vi "Begin.vi"(8 "error in":errorcluster) -> (0 "error out":errorcluster)   [LabVIEW 2015]
doc: "Called before other user functions, this VI is expected to open initial I/O refnums, load in file data, and do all program initialization. Notice that the <B>error out</B> terminal is simply used for data flow. Wiring it to other structures or subVIs ensures that this VI runs first."
uses:
  <vilib>/Rock Robotics/WPI/SafetyOutput/WPI_SafetyOutputConfigMenu.ctl
  <vilib>/Rock Robotics/WPI/DriverStation/WPI_DriverStationRobotMode2.ctl
  <vilib>/Rock Robotics/WPI/Joystick/WPI_JoystickDeviceEnum.ctl
  <vilib>/Rock Robotics/SystemInterfaces/DIO/FPGA_DIOPWMChannel.ctl
  <vilib>/Rock Robotics/SystemInterfaces/AI/FPGA_AIGyroChannel.ctl
  Robot Global Data.vi
  <vilib>/Rock Robotics/Network Tables/NT Write String Array.vi
  <vilib>/Rock Robotics/WPI/MotorControl/WPI_MotorControlOpen Talon.vi
  <vilib>/Rock Robotics/WPI/RobotDrive/WPI_RobotDriveOpen4MotorWithExistingMotors.vi
  <vilib>/Rock Robotics/WPI/MotorControl/WPI_MotorControlOpen VictorSP.vi
  <vilib>/Rock Robotics/WPI/RobotDrive/WPI_RobotDriveOpen2MotorWithExistingMotors.vi
  <vilib>/Rock Robotics/WPI/Switch/WPI_SwitchOpenLimit.vi
  <vilib>/Rock Robotics/WPI/MotorControl/WPI_MotorControlOpen SPARK.vi
  <vilib>/Rock Robotics/WPI/MotorControl/WPI_MotorControlOpenCANTalonSRX.vi
  <vilib>/Rock Robotics/WPI/Gyro/WPI_GyroAnalogOpen.vi
  <vilib>/Rock Robotics/Network Tables/NT Write String.vi
  <vilib>/Rock Robotics/SystemInterfaces/spilib/spi_bus.ctl
  <vilib>/Rock Robotics/SystemInterfaces/DIO/FPGA_DIOChannel.ctl
  <vilib>/Rock Robotics/WPI/CAN/TalonSRX/WPI_CANTalonSRX_APIControlMode.ctl
  ADI MXP IMU/ADI MXP IMU/FRC ADI MXP IMU.lvlib
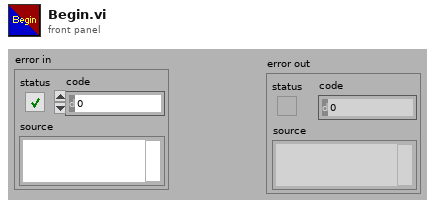
[diagram p1: front panel]
types:
  T1 = typedef "WPI_JoystickDeviceEnum.ctl" = enum16{"USB 0", "USB 1", "USB 2", "USB 3", "USB 4", "USB 5"}
  T2 = typedef "WPI_DriverStationRobotMode2.ctl" = enum16{"Autonomous Disabled", "Autonomous Enabled", "Teleop Disabled", "Teleop Enabled", "Disconnected", "Finish", "Test Disabled", "Test Enabled", "Emergency Stopped"}
  T3 = typedef "WPI_SafetyOutputConfigMenu.ctl" = enum16{"Enable", "Disable"}
  T4 = typedef "FPGA_DIOPWMChannel.ctl" = enum8{"PWM 0", "PWM 1", "PWM 2", "PWM 3", "PWM 4", "PWM 5", "PWM 6", "PWM 7", "PWM 8", "PWM 9", "PWM MXP 0", "PWM MXP 1", "PWM MXP 2", "PWM MXP 3", "PWM MXP 4", "PWM MXP 5", "PWM MXP 6", "PWM MXP 7", "PWM MXP 8", "PWM MXP 9", "Invalid"}
  T5 = typedef "WPI_MotorControlDeviceRef.ctl" = cluster{"DeviceStatus":errorcluster, "Type":T6, "PWM":cluster{"PWM Channel":T4, "DeadBand":T7}, "CAN":cluster{"Device Number":u8, "Control Mode":T8, "Semaphore":T9, "Max Vout":dbl, "TalonSRX Control Mode":T10}, "Invert":bool}
  T6 = typedef "WPI_MotorControlType.ctl" = enum16{"PWM", "CAN", "CANTalonSRX"}
  T7 = typedef "WPI_PWMDeadband.ctl" = cluster{"Name":string, "maxPositivePwm":i32, "minPositivePwm":i32, "centerPwm":i32, "maxNegativePwm":i32, "minNegativePwm":i32, "angularRange":u16}
  T8 = typedef "WPI_CANJaguar_ControlMode.ctl" = enum8{"Percent VBus", "Current", "Speed", "Position", "Voltage"}
  T9 = typedef "Semaphore RefNum" = refnum<k1>
  T10 = typedef "WPI_CANTalonSRX_APIControlMode.ctl" = enum8{"Percent VBus", "Speed", "Position", "Slave", "Unchanged / Invalid", "Voltage Compensation", "Current", "Motion Profile"}
  T11 = typedef "WPI_RobotDriveDevRef.ctl" = cluster{"DevStatus":errorcluster, "Motors[]":T5[], "Square Inputs":bool, "Max Output":dbl}
  T12 = typedef "WPI_JoystickDevRef.ctl" = cluster{"Device":T1}
  T13 = typedef "FPGA_DIOChannel.ctl" = enum8{"DIO 0", "DIO 1", "DIO 2", "DIO 3", "DIO 4", "DIO 5", "DIO 6", "DIO 7", "DIO 8", "DIO 9", "DIO MXP 0", "DIO MXP 1", "DIO MXP 2", "DIO MXP 3", "DIO MXP 4", "DIO MXP 5", "DIO MXP 6", "DIO MXP 7", "DIO MXP 8", "DIO MXP 9", "DIO MXP 10", "DIO MXP 11", "DIO MXP 12", "DIO MXP 13", "DIO MXP 14", "DIO MXP 15", "Invalid"}
  T14 = typedef "spi_bus.ctl" = enum16{"SPI On-Board, CS0", "SPI On-Board, CS1", "SPI On-Board, CS2", "SPI On-Board, CS3", "SPI MXP", "Invalid"}
  T15 = typedef "FPGA_AIGyroChannel.ctl" = enum8{"AI 0", "AI 1", "Invalid"}
  T16 = typedef "WPI_DigitalInputDevRef.ctl" = cluster{"DevStatus":errorcluster, "DIO Channel":T13}
  T17 = typedef "WPI_SwitchDevRef.ctl" = cluster{"DevStatus":errorcluster, "DIO Channel":T13, "CntIndex":T18, "Normally Closed":bool}
  T18 = typedef "FPGA_CounterCtrSystemIndex.ctl" = enum8{"Ctr 0", "Ctr 1", "Ctr 2", "Ctr 3", "Ctr 4", "Ctr 5", "Ctr 6", "Ctr 7", "Invalid"}
  T19 = typedef "FRC ADI MXP IMU.lvlib/WPI_AnalogDevicesIMUInterruptDevRef.ctl" = cluster{"SimpleGyroDevRef":T20, "InterruptRef":T21}
  T20 = typedef "FRC ADI MXP IMU.lvlib/WPI_AnalogDevicesIMUDevRef.ctl" = cluster{"DevStatus":errorcluster, "Handle":i32, "SPI Bus":T14, "Device Found":bool, "Sample Rate":dbl, "Device Ready":bool, "Yaw Axis":enum16{"X", "Y", "Z"}, "AHRS Algorithm":enum16{"Complementary", "Madgwick"}}
  T21 = typedef "WPI_InterruptRef.ctl" = cluster{"DevStatus":errorcluster, "InterruptIndex":T22}
  T22 = typedef "FPGA_InterruptIndex.ctl" = enum8{"0", "1", "2", "3", "4", "5", "6", "7", "Invalid"}
  T23 = typedef "WPI_GyroDevRef.ctl" = cluster{"DevStatus":errorcluster, "Analog Channel":T24, "Offset":dbl, "Gain (VoltsPerDegree/Second)":dbl, "Gyro Type":enum16{"Analog", "XRS450"}, "Handle":i32, "SPI Bus":T14, "Device Found":bool, "Sample Rate":dbl, "Calibrate On Open":bool}
  T24 = typedef "FPGA_AIChannel.ctl" = enum8{"AI 0", "AI 1", "AI 2", "AI 3", "AI MXP 0", "AI MXP 1", "AI MXP 2", "AI MXP 3", "Invalid"}
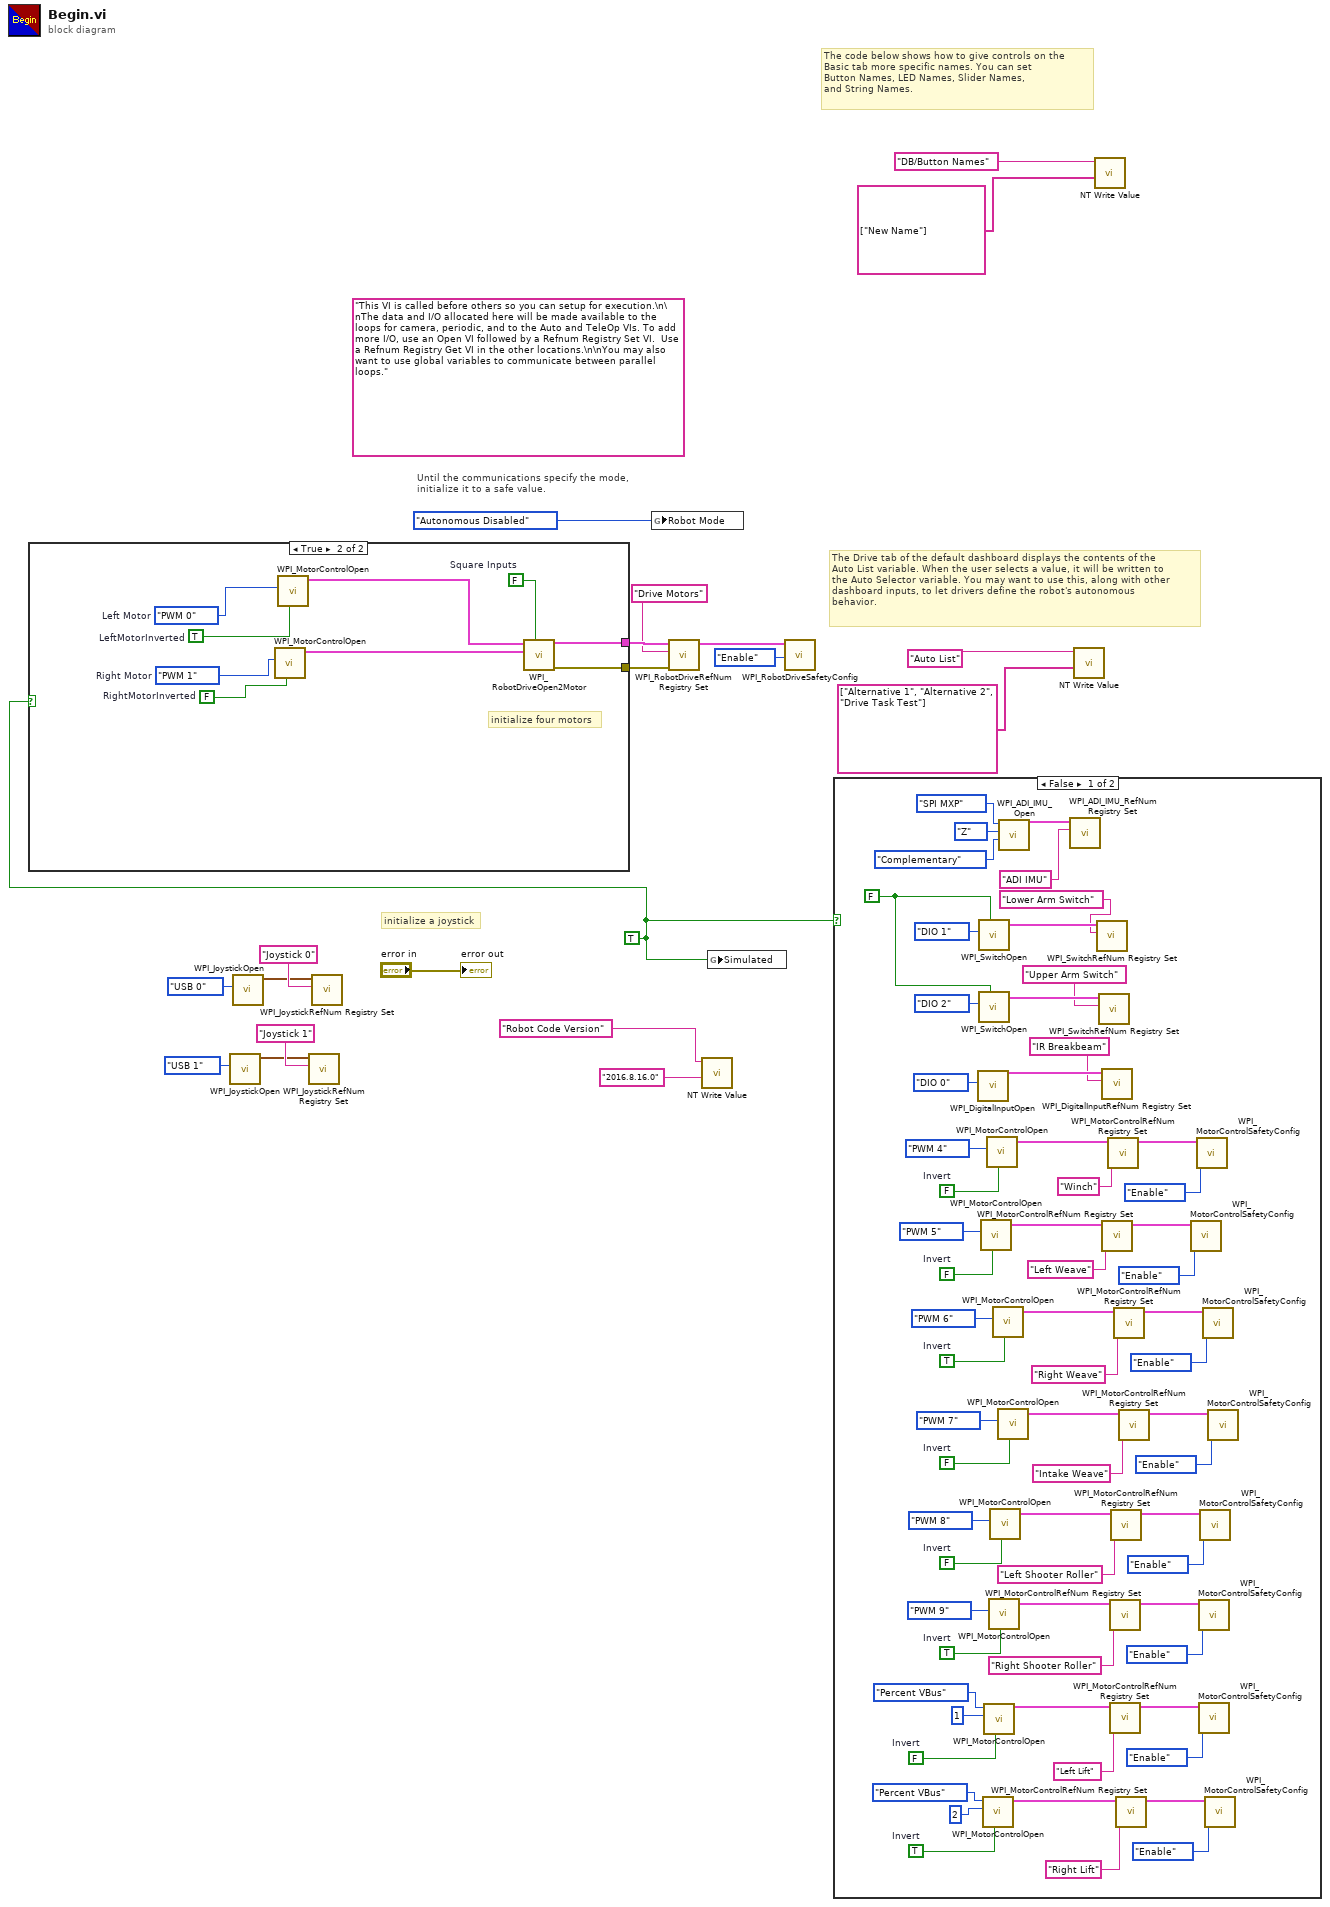
[diagram p0: block diagram]
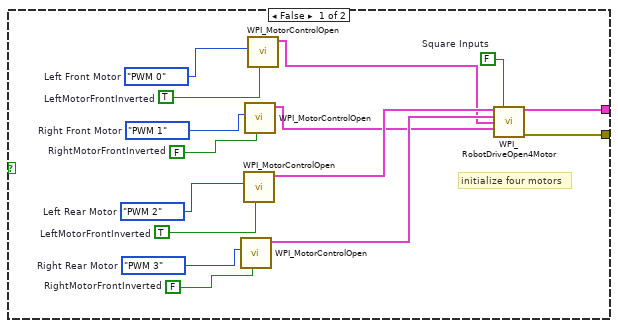
[diagram p2: hidden frame]
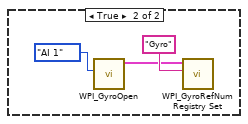
[diagram p3: hidden frame]
diagram:
  w1 = TRUE
  (unwired) "This VI is called before others so you can setup for execution.\n\nThe data and I/O allocated here will be made available to the loops for camera, periodic, and to the Auto and TeleOp VIs. To add more I/O, use an Open VI followed by a Refnum Registry Set VI.  Use a Refnum Registry Get VI in the other locations.\n\nYou may also want to use global variables to communicate between parallel loops."
  # "The Drive tab of the default dashboard displays the contents of the\nAuto List variable. When the user selects a value, it will be written to\nthe Auto Selector variable. You may want to use this, along with other\ndashboard inputs, to let drivers define the robot's autonomous\nbehavior."
  # "The code below shows how to give controls on the\nBasic tab more specific names. You can set\nButton Names, LED Names, Slider Names,\nand String Names."
  # "initialize a joystick"
  # "Until the communications specify the mode,\ninitialize it to a safe value."
  n1 = case shown="True" w1 {
    tunnel: [w35 w36] -> w20
    tunnel: [w34 w37] -> w18
    frame False {
      w27 = FPGA_DIOPWMChannel."PWM 3"  # Right Rear Motor
      w26 = FPGA_DIOPWMChannel."PWM 2"  # Left Rear Motor
      w25 = TRUE  # LeftMotorFrontInverted
      w28 = FALSE  # RightMotorFrontInverted
      w29 = FALSE  # Square Inputs
      w32 = FPGA_DIOPWMChannel."PWM 1"  # Right Front Motor
      w31 = FPGA_DIOPWMChannel."PWM 0"  # Left Front Motor
      w30 = TRUE  # LeftMotorFrontInverted
      w33 = FALSE  # RightMotorFrontInverted
      # "initialize four motors"
      n2 = call-poly <vilib>:"WPI_MotorControlOpen.vi"("Invert"=w28, "PWM Channel"=w27) -> ("MotorControlDeviceRef"=w23:T5)  [unwired: 8 in, 1 out]
      n3 = call-poly <vilib>:"WPI_MotorControlOpen.vi"("Invert"=w25, "PWM Channel"=w26) -> ("MotorControlDeviceRef"=w24:T5)  [unwired: 8 in, 1 out]
      n4 = call-poly <vilib>:"WPI_MotorControlOpen.vi"("Invert"=w33, "PWM Channel"=w32) -> ("MotorControlDeviceRef"=w21:T5)  [unwired: 8 in, 1 out]
      n5 = call-poly <vilib>:"WPI_MotorControlOpen.vi"("Invert"=w30, "PWM Channel"=w31) -> ("MotorControlDeviceRef"=w22:T5)  [unwired: 8 in, 1 out]
      n6 = call-poly <vilib>:"WPI_RobotDriveOpen4Motor.vi"("Rear Left Motor Dev Ref"=w24, "Square Inputs"=w29, "Rear Right Motor Dev Ref"=w23, "Front Left Motor Dev Ref"=w22, "Front Right Motor Dev Ref"=w21) -> ("RobotDriveDevRef"=w35:T11, "error out"=w34:errorcluster)  [unwired: 9 in]
    }
    frame True {
      w40 = FALSE  # Square Inputs
      w43 = FPGA_DIOPWMChannel."PWM 1"  # Right Motor
      w42 = FPGA_DIOPWMChannel."PWM 0"  # Left Motor
      w41 = TRUE  # LeftMotorInverted
      w44 = FALSE  # RightMotorInverted
      # "initialize four motors"
      n7 = call-poly <vilib>:"WPI_MotorControlOpen.vi"("Invert"=w44, "PWM Channel"=w43) -> ("MotorControlDeviceRef"=w38:T5)  [unwired: 8 in, 1 out]
      n8 = call-poly <vilib>:"WPI_MotorControlOpen.vi"("Invert"=w41, "PWM Channel"=w42) -> ("MotorControlDeviceRef"=w39:T5)  [unwired: 8 in, 1 out]
      n9 = call-poly <vilib>:"WPI_RobotDriveOpen2Motor.vi"("Square Inputs"=w40, "Right Motor Dev Ref"=w38, "Left Motor Dev Ref"=w39) -> ("error out"=w37:errorcluster, "RobotDriveDevRef"=w36:T11)  [unwired: 7 in]
    }
  }
  n10 = call <vilib>:"WPI_JoystickOpen.vi"("JoystickDevice"=WPI_JoystickDeviceEnum."USB 1") -> ("JoystickDevRef"=w5:T12)  [unwired: 10 in]
  n11 = call <vilib>:"WPI_JoystickOpen.vi"("JoystickDevice"=WPI_JoystickDeviceEnum."USB 0") -> ("JoystickDevRef"=w13:T12)  [unwired: 10 in]
  n12 = call <vilib>:"WPI_JoystickRefNum Registry Set.vi"("refnum name"="Joystick 1", "JoystickDevRef"=w5) -> ()  [unwired: 8 in, 2 out]
  n13 = call <vilib>:"WPI_JoystickRefNum Registry Set.vi"("refnum name"="Joystick 0", "JoystickDevRef"=w13) -> ()  [unwired: 8 in, 2 out]
  n14 = global write "Robot Global Data.vi" "Robot Mode"(WPI_DriverStationRobotMode2."Autonomous Disabled" ("Robot Mode")) -> ()
  n15 = call <vilib>:"WPI_RobotDriveRefNum Registry Set.vi"("error in (no error)"=w18, "refnum name"="Drive Motors", "RobotDriveDevRef"=w20) -> ("RobotDriveDevRef"=w17:T11)  [unwired: 1 in, 7 out]
  n16 = call-poly <vilib>:"NT Write Value.vi"("String"="2016.8.16.0", "Name"="Robot Code Version") -> ()  [unwired: 9 in, 1 out]
  n17 = global write "Robot Global Data.vi" "Simulated"(w1) -> ()
  n18 = call <vilib>:"WPI_RobotDriveSafetyConfig.vi"("mode"=WPI_SafetyOutputConfigMenu."Enable", "RobotDriveDevRef"=w17) -> ()  [unwired: 8 in, 2 out]
  n19 = case shown="False" w1 {
    frame False {
      w45 = FALSE  # Invert
      w46 = TRUE  # Invert
      w47 = FALSE  # Invert
      w48 = FALSE  # Invert
      w49 = TRUE  # Invert
      w50 = FALSE  # Invert
      w51 = FALSE  # Invert
      w52 = TRUE  # Invert
      w101 = FALSE ("Normally Closed")
      n20 = call <vilib>:"WPI_DigitalInputOpen.vi"("DIO Channel"=FPGA_DIOChannel."DIO 0") -> ("DigitalInputDevRef"=w97:T16)  [unwired: 9 in, 1 out]
      n21 = call-poly <vilib>:"WPI_SwitchOpen.vi"("Normally Closed"=w101, "DIO Channel"=FPGA_DIOChannel."DIO 1") -> ("SwitchDevRef"=w102:T17)  [unwired: 8 in, 1 out]
      n22 = call-poly <vilib>:"WPI_SwitchOpen.vi"("Normally Closed"=w101, "DIO Channel"=FPGA_DIOChannel."DIO 2") -> ("SwitchDevRef"=w100:T17)  [unwired: 8 in, 1 out]
      n23 = call-poly <vilib>:"WPI_MotorControlOpen.vi"("Invert"=w50, "PWM Channel"=FPGA_DIOPWMChannel."PWM 5") -> ("MotorControlDeviceRef"=w93:T5)  [unwired: 8 in, 1 out]
      n24 = call-poly <vilib>:"WPI_MotorControlOpen.vi"("Invert"=w46, "Device Number"=u8 2, "Control Mode"=WPI_CANTalonSRX_APIControlMode."Percent VBus") -> ("MotorControlDeviceRef"=w60:T5)  [unwired: 7 in, 1 out]
      n25 = call-poly <vilib>:"WPI_MotorControlOpen.vi"("Invert"=w47, "Device Number"=u8 1, "Control Mode"=WPI_CANTalonSRX_APIControlMode."Percent VBus") -> ("MotorControlDeviceRef"=w63:T5)  [unwired: 7 in, 1 out]
      n26 = call-poly <vilib>:"WPI_MotorControlOpen.vi"("Invert"=w45, "PWM Channel"=FPGA_DIOPWMChannel."PWM 4") -> ("MotorControlDeviceRef"=w56:T5)  [unwired: 8 in, 1 out]
      n27 = call-poly <vilib>:"WPI_MotorControlOpen.vi"("Invert"=w52, "PWM Channel"=FPGA_DIOPWMChannel."PWM 9") -> ("MotorControlDeviceRef"=w73:T5)  [unwired: 8 in, 1 out]
      n28 = call-poly <vilib>:"WPI_MotorControlOpen.vi"("Invert"=w51, "PWM Channel"=FPGA_DIOPWMChannel."PWM 8") -> ("MotorControlDeviceRef"=w78:T5)  [unwired: 8 in, 1 out]
      n29 = call-poly <vilib>:"WPI_MotorControlOpen.vi"("Invert"=w49, "PWM Channel"=FPGA_DIOPWMChannel."PWM 6") -> ("MotorControlDeviceRef"=w88:T5)  [unwired: 8 in, 1 out]
      n30 = call-poly <vilib>:"WPI_MotorControlOpen.vi"("Invert"=w48, "PWM Channel"=FPGA_DIOPWMChannel."PWM 7") -> ("MotorControlDeviceRef"=w83:T5)  [unwired: 8 in, 1 out]
      n31 = call "WPI_ADI_IMU_Open.vi"("AHRS Algorithm"=enum16{"Complementary", "Madgwick"}."Complementary", "Yaw Axis"=enum16{"X", "Y", "Z"}."Z", "SPI Chip Select"=spi_bus."SPI MXP") -> ("ADI IMU Interrupt DevRef"=w106:T19)  [unwired: 7 in, 1 out]
      n32 = call "WPI_ADI_IMU_RefNum Registry Set.vi"("refnum name"="ADI IMU", "ADI IMU Interrupt DevRef"=w106) -> ()  [unwired: 8 in, 2 out]
      n33 = call <vilib>:"WPI_SwitchRefNum Registry Set.vi"("refnum name"="Lower Arm Switch", "SwitchDevRef"=w102) -> ()  [unwired: 8 in, 2 out]
      n34 = call <vilib>:"WPI_SwitchRefNum Registry Set.vi"("refnum name"="Upper Arm Switch", "SwitchDevRef"=w100) -> ()  [unwired: 8 in, 2 out]
      n35 = call <vilib>:"WPI_DigitalInputRefNum Registry Set.vi"("refnum name"="IR Breakbeam", "DigitalInputDevRef"=w97) -> ()  [unwired: 8 in, 2 out]
      n36 = call <vilib>:"WPI_MotorControlRefNum Registry Set.vi"("refnum name"="Left Weave", "MotorControlDevRef"=w93) -> ("MotorControlDevRef"=w92:T5)  [unwired: 8 in, 1 out]
      n37 = call <vilib>:"WPI_MotorControlRefNum Registry Set.vi"("refnum name"="Winch", "MotorControlDevRef"=w56) -> ("MotorControlDevRef"=w55:T5)  [unwired: 8 in, 1 out]
      n38 = call <vilib>:"WPI_MotorControlRefNum Registry Set.vi"("refnum name"="Right Shooter Roller", "MotorControlDevRef"=w73) -> ("MotorControlDevRef"=w72:T5)  [unwired: 8 in, 1 out]
      n39 = call <vilib>:"WPI_MotorControlRefNum Registry Set.vi"("refnum name"="Left Lift", "MotorControlDevRef"=w63) -> ("MotorControlDevRef"=w65:T5)  [unwired: 8 in, 1 out]
      n40 = call <vilib>:"WPI_MotorControlRefNum Registry Set.vi"("refnum name"="Left Shooter Roller", "MotorControlDevRef"=w78) -> ("MotorControlDevRef"=w77:T5)  [unwired: 8 in, 1 out]
      n41 = call <vilib>:"WPI_MotorControlRefNum Registry Set.vi"("refnum name"="Right Weave", "MotorControlDevRef"=w88) -> ("MotorControlDevRef"=w87:T5)  [unwired: 8 in, 1 out]
      n42 = call <vilib>:"WPI_MotorControlRefNum Registry Set.vi"("refnum name"="Right Lift", "MotorControlDevRef"=w60) -> ("MotorControlDevRef"=w62:T5)  [unwired: 8 in, 1 out]
      n43 = call <vilib>:"WPI_MotorControlRefNum Registry Set.vi"("refnum name"="Intake Weave", "MotorControlDevRef"=w83) -> ("MotorControlDevRef"=w82:T5)  [unwired: 8 in, 1 out]
      n44 = call <vilib>:"WPI_MotorControlSafetyConfig.vi"("mode"=WPI_SafetyOutputConfigMenu."Enable", "MotorControlDevRef"=w92) -> ()  [unwired: 8 in, 2 out]
      n45 = call <vilib>:"WPI_MotorControlSafetyConfig.vi"("mode"=WPI_SafetyOutputConfigMenu."Enable", "MotorControlDevRef"=w55) -> ()  [unwired: 8 in, 2 out]
      n46 = call <vilib>:"WPI_MotorControlSafetyConfig.vi"("mode"=WPI_SafetyOutputConfigMenu."Enable", "MotorControlDevRef"=w72) -> ()  [unwired: 8 in, 2 out]
      n47 = call <vilib>:"WPI_MotorControlSafetyConfig.vi"("mode"=WPI_SafetyOutputConfigMenu."Enable", "MotorControlDevRef"=w65) -> ()  [unwired: 8 in, 2 out]
      n48 = call <vilib>:"WPI_MotorControlSafetyConfig.vi"("mode"=WPI_SafetyOutputConfigMenu."Enable", "MotorControlDevRef"=w77) -> ()  [unwired: 8 in, 2 out]
      n49 = call <vilib>:"WPI_MotorControlSafetyConfig.vi"("mode"=WPI_SafetyOutputConfigMenu."Enable", "MotorControlDevRef"=w87) -> ()  [unwired: 8 in, 2 out]
      n50 = call <vilib>:"WPI_MotorControlSafetyConfig.vi"("mode"=WPI_SafetyOutputConfigMenu."Enable", "MotorControlDevRef"=w62) -> ()  [unwired: 8 in, 2 out]
      n51 = call <vilib>:"WPI_MotorControlSafetyConfig.vi"("mode"=WPI_SafetyOutputConfigMenu."Enable", "MotorControlDevRef"=w82) -> ()  [unwired: 8 in, 2 out]
    }
    frame True {
      n52 = call-poly <vilib>:"WPI_GyroOpen.vi"("Analog Channel"=FPGA_AIGyroChannel."AI 1") -> ("GyroDevRef"=w110:T23)  [unwired: 8 in, 2 out]
      n53 = call <vilib>:"WPI_GyroRefNum Registry Set.vi"("refnum name"="Gyro", "GyroDevRef"=w110) -> ()  [unwired: 8 in, 2 out]
    }
  }
  n54 = call-poly <vilib>:"NT Write Value.vi"("String Array"=string[] ["Alternative 1", "Alternative 2", "Drive Task Test"], "Name"="Auto List") -> ()  [unwired: 9 in, 1 out]
  n55 = call-poly <vilib>:"NT Write Value.vi"("String Array"=string[] ["New Name"], "Name"="DB/Button Names") -> ()  [unwired: 9 in, 1 out]
  "error out" <- "error in"
